vi "KE6221 -- Get Arb Loc0 Waveform Points.vi"(0 "Resource In":refnum<visa-resource-name>, 1 "Check For SCPI Errors? (T)":bool=TRUE, 11 "error in (no error)":errorcluster, 13 "Timeout (10000 ms)":u32=10000) -> (4 "Resource Out (dupl)":refnum<visa-resource-name>, 6 "Num Points":u32, 8 "Arb Waveform Points":T1[](array[typedef]) min=-1.0 max=1.0 format="%.3f", 15 "error out":errorcluster)   [LabVIEW 2019, in "Keithley 622x.lvlib"]
uses:
  Keithley 622x.lvlib
  Typedefs/KE6221 -- Wave Arb Point.ctl
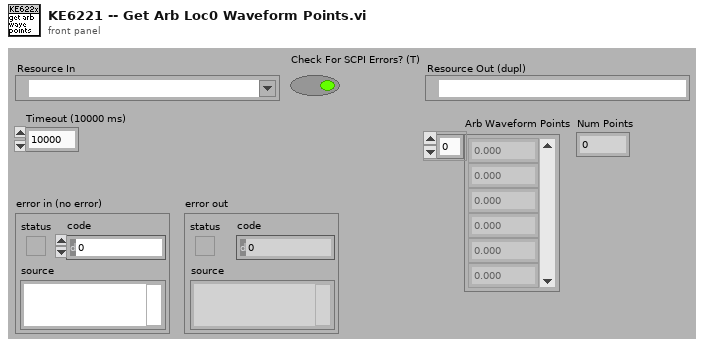
[diagram p1: front panel]
types:
  T1 = typedef "Keithley 622x.lvlib/KE6221 -- Wave Arb Point.ctl" = dbl
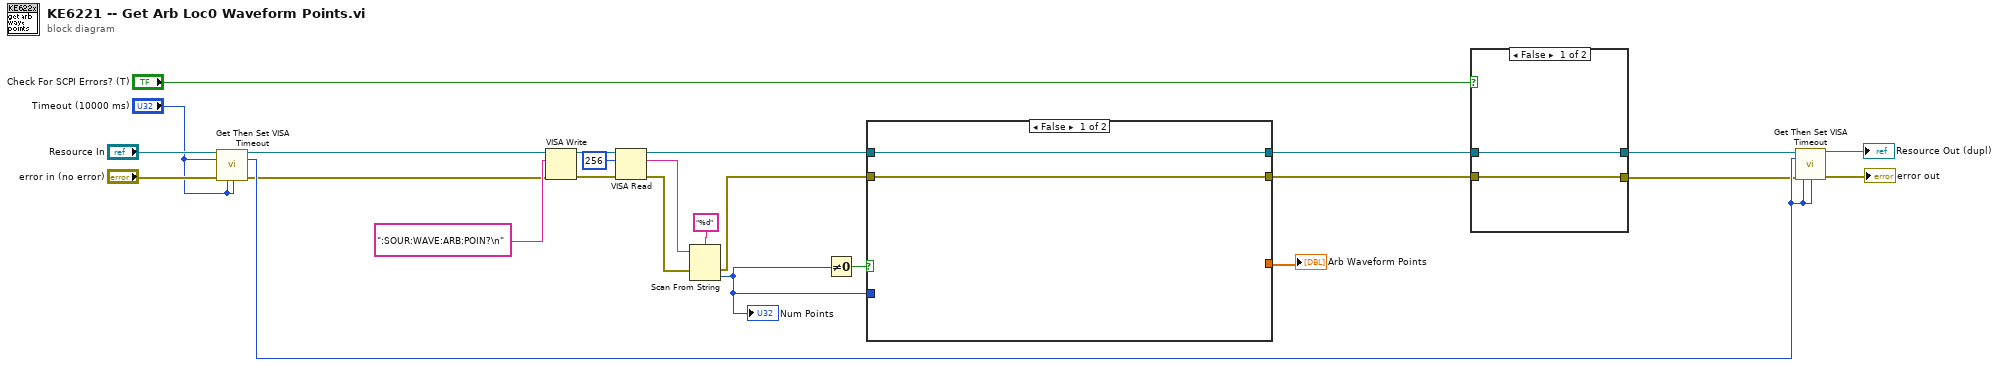
[diagram p0: block diagram]
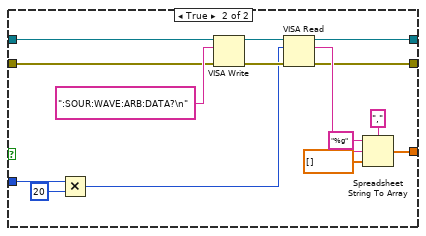
[diagram p2: hidden frame]
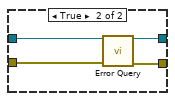
[diagram p3: hidden frame]
diagram:
  n1 = call "Get Then Set VISA Timeout.vi"("VISA Resource Name In"="Resource In", "New Timeout (msecs)"="Timeout (10000 ms)", "error in (no error)"="error in (no error)", "Max Timeout (300 secs)"="Timeout (10000 ms)", "Min Timeout (3 secs)"="Timeout (10000 ms)") -> ("VISA Resource Name Out (dupl)"=w4:refnum<visa-resource-name>, "Old Timeout (msecs)"=w8:u32, "error out"=w3:errorcluster)  [unwired: 7 in, 1 out]
  n2 = VISA Write(VISA resource name=w4, write buffer=":SOUR:WAVE:ARB:POIN?\n" ("format string"), error in (no error)=w3) -> (VISA resource name out=w24:refnum<visa-resource-name>, error out=w23:errorcluster)  [unwired: 1 out]
  n3 = VISA Read(VISA resource name=w24, byte count=u32 256, error in (no error)=w23) -> (VISA resource name out=w16:refnum<visa-resource-name>, read buffer=w19:string, error out=w21:errorcluster)  [unwired: 1 out]
  n4 = Scan From String(format string="%d", input string=w19, error in=w21) -> (error out=w17:errorcluster, output 1=w15:u32)  [unwired: 2 in, 2 out]
  "Num Points" <- w15
  n5 = Not Equal To 0?(x=w15) -> (x != 0?=w18:bool)
  n6 = case shown="False" w18 {
    tunnel: w17 -> [w26 w39]
    tunnel: w16 -> [w27 w38]
    tunnel: w15 -> [_ w37]
    tunnel: [_ w30] -> w14
    tunnel: [w26 w29] -> w1
    tunnel: [w27 w28] -> w2
    frame False {
    }
    frame True {
      n7 = Multiply(x=w37, y=u32 20) -> (x*y=w35:u32)
      n8 = VISA Write(VISA resource name=w38, write buffer=":SOUR:WAVE:ARB:DATA?\n" ("format string"), error in (no error)=w39) -> (VISA resource name out=w41:refnum<visa-resource-name>, error out=w40:errorcluster)  [unwired: 1 out]
      n9 = VISA Read(VISA resource name=w41, byte count=w35, error in (no error)=w40) -> (VISA resource name out=w28:refnum<visa-resource-name>, read buffer=w34:string, error out=w29:errorcluster)  [unwired: 1 out]
      n10 = Spreadsheet String To Array(delimiter (Tab)=",", format string="%g", spreadsheet string=w34, array type (2D Dbl)=dbl[] []) -> (array=w30:dbl[])
    }
  }
  "Arb Waveform Points" <- w14
  n11 = case shown="False" "Check For SCPI Errors? (T)" {
    tunnel: w2 -> [w44 w48]
    tunnel: w1 -> [w43 w47]
    tunnel: [w43 w46] -> w5
    tunnel: [w44 w45] -> w6
    frame False {
    }
    frame True {
      n12 = call "Error Query.vi"("VISA Resource In"=w48, "error in (no error)"=w47) -> ("VISA Resource Out (dupl)"=w45:refnum<visa-resource-name>, "error out"=w46:errorcluster)  [unwired: 10 in, 2 out]
    }
  }
  n13 = call "Get Then Set VISA Timeout.vi"("VISA Resource Name In"=w6, "New Timeout (msecs)"=w8, "error in (no error)"=w5, "Max Timeout (300 secs)"=w8, "Min Timeout (3 secs)"=w8) -> ("VISA Resource Name Out (dupl)"=→"Resource Out (dupl)":refnum<visa-resource-name>, "error out"=→"error out":errorcluster)  [unwired: 7 in, 2 out]
